vi "novo_config_adq.vi"() -> ()   [LabVIEW 2019]
uses:
  Aplicacao_atual_global_adq.vi
  <vilib>/Utility/file.llb/Write Delimited Spreadsheet (DBL).vi
panel:
  in  "SKM-AI-KF_COR":bool
  in  "SKM-FIC-KF_COR":bool
  in  "SKM-FI-WF":bool
  in  "JG":bool
  in  "JK":bool
  in  "JW":bool
  out "path":path
  in  "SALVAR":bool
  in  "Pfundo":bool
  in  "P4":bool
  in  "P3":bool
  in  "P2":bool
  in  "P1":bool
  in  "C4-M":bool
  in  "C4-J":bool
  in  "C3-J":bool
  in  "C3-M":bool
  in  "C2-J":bool
  in  "C2-M":bool
  in  "C1-J":bool
  in  "C1-M":bool
  # "NOVA CONFIGURACAO PARA O ADQUIRI"
  # "Selecione todos os Instrumento/Valores que deseja trabalhar e salvar no adquiri"
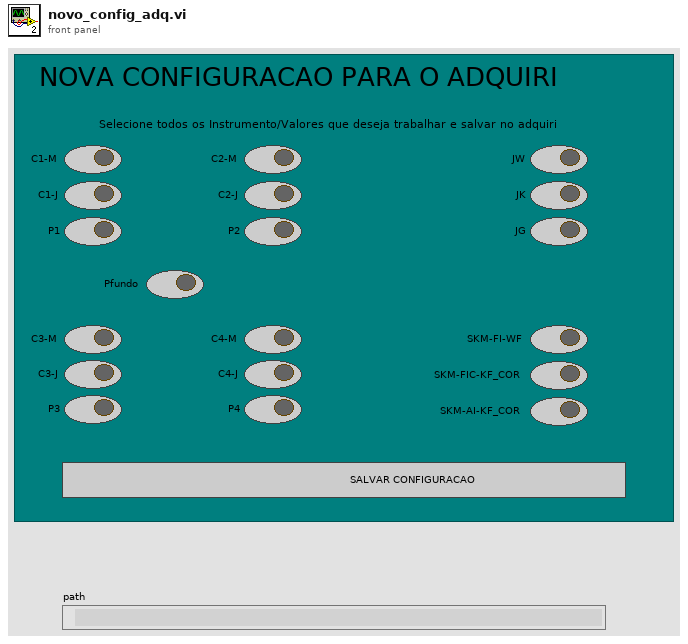
[diagram p1: front panel]
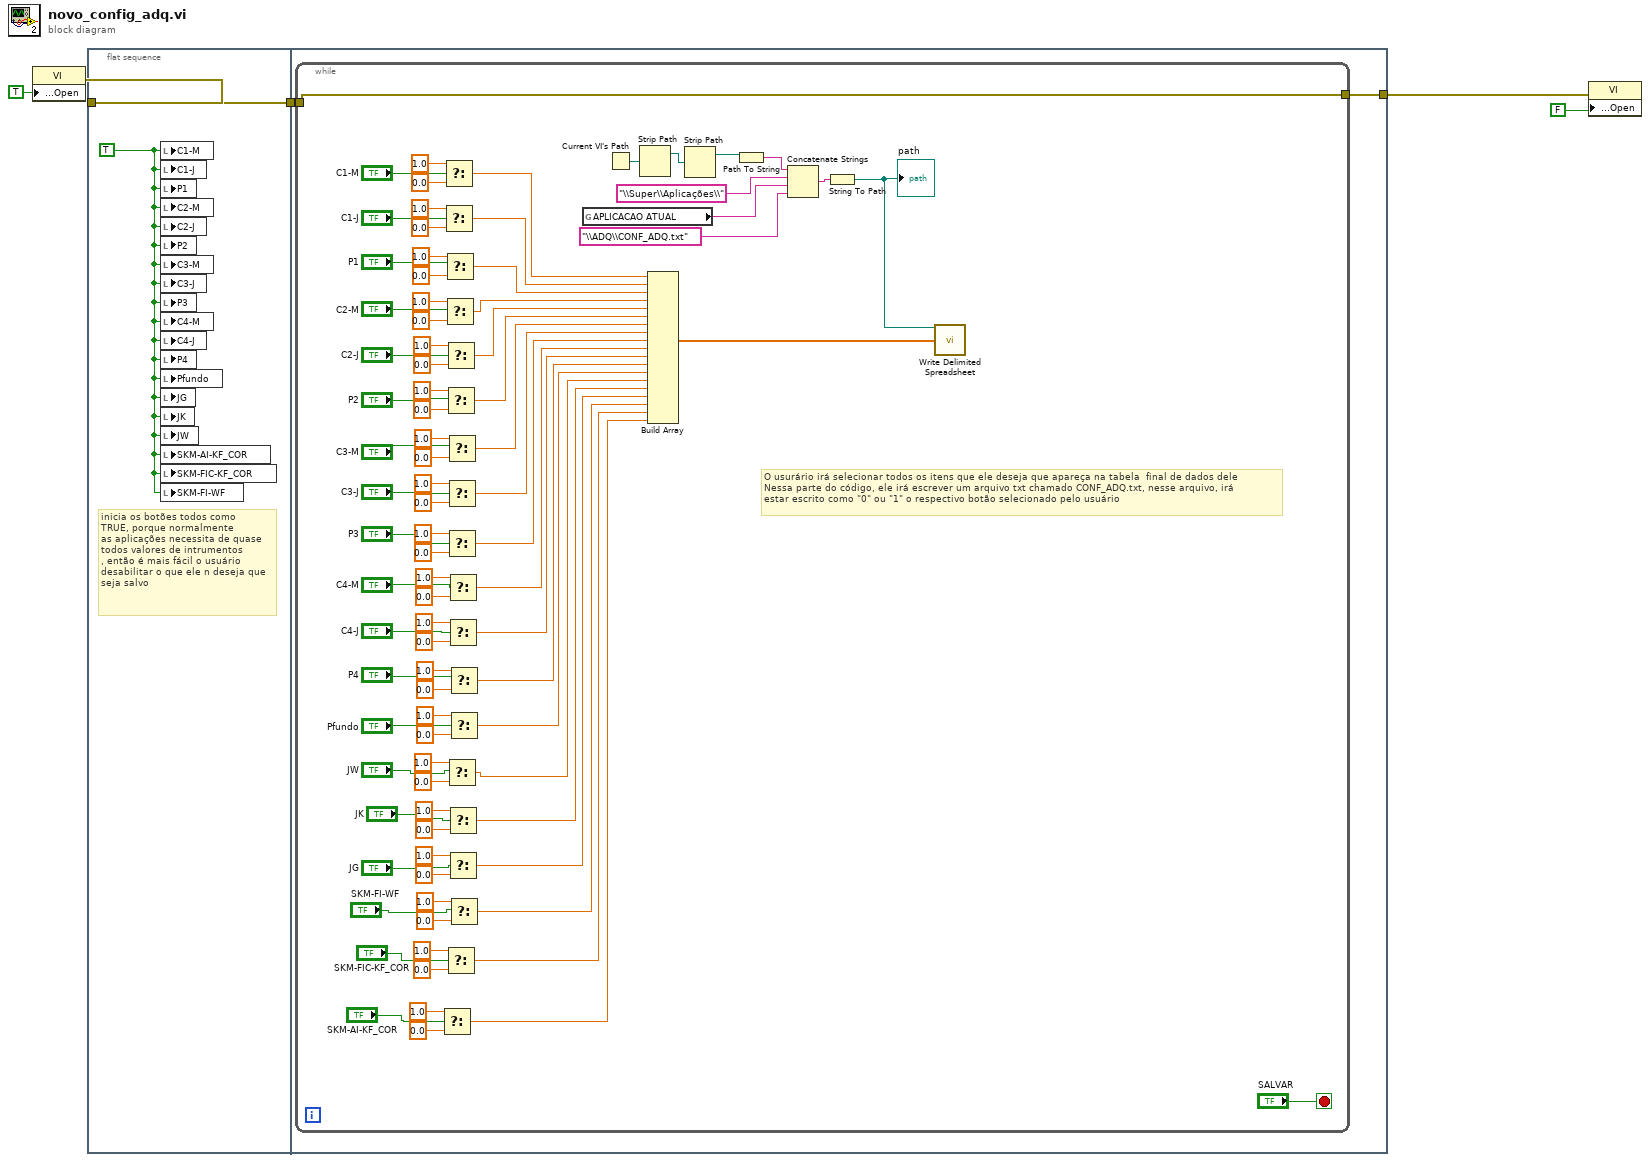
[diagram p0: block diagram]
diagram:
  n1 = property class="VI"("Front Panel.Open"=TRUE ("Front Panel Window:Open")) -> (error out=w3:errorcluster)  [unwired: 2 in, 1 out]
  n2 = flat-sequence {
    tunnel: w3 -> [w7]
    tunnel: [w7] -> w2
    tunnel: w2 -> [w8]
    tunnel: [w9] -> w5
    frame #0 {
      w6 = TRUE ("C1-M")
      # "inicia os botões todos como\nTRUE, porque normalmente\nas aplicações necessita de quase\ntodos valores de intrumentos\n, então é mais fácil o usuário \ndesabilitar o que ele n deseja que\nseja salvo"
      n3 = local write "C1-M"(w6) -> ()
      n4 = local write "C1-J"(w6) -> ()
      n5 = local write "P1"(w6) -> ()
      n6 = local write "C2-M"(w6) -> ()
      n7 = local write "C2-J"(w6) -> ()
      n8 = local write "P2"(w6) -> ()
      n9 = local write "C3-M"(w6) -> ()
      n10 = local write "C3-J"(w6) -> ()
      n11 = local write "P3"(w6) -> ()
      n12 = local write "C4-M"(w6) -> ()
      n13 = local write "C4-J"(w6) -> ()
      n14 = local write "P4"(w6) -> ()
      n15 = local write "Pfundo"(w6) -> ()
      n16 = local write "JG"(w6) -> ()
      n17 = local write "JK"(w6) -> ()
      n18 = local write "JW"(w6) -> ()
      n19 = local write "SKM-AI-KF_COR"(w6) -> ()
      n20 = local write "SKM-FIC-KF_COR"(w6) -> ()
      n21 = local write "SKM-FI-WF"(w6) -> ()
    }
    frame #1 {
      n22 = while {
        tunnel: w8 -> [w24]
        tunnel: [w24] -> w9
        stop <- "SALVAR" stop-if-true
        # "O usurário irá selecionar todos os itens que ele deseja que apareça na tabela  final de dados dele\nNessa parte do código, ele irá escrever um arquivo txt chamado CONF_ADQ.txt, nesse arquivo, irá \nestar escrito como \"0\" ou \"1\" o respectivo botão selecionado pelo usuário"
        n23 = Select(t=1.0, s="SKM-AI-KF_COR", f=0.0) -> (s? t:f=w10:dbl)
        n24 = Select(t=1.0, s="C1-M", f=0.0) -> (s? t:f=w66:dbl)
        n25 = Select(t=1.0, s="C1-J", f=0.0) -> (s? t:f=w65:dbl)
        n26 = Select(t=1.0, s="P1", f=0.0) -> (s? t:f=w64:dbl)
        n27 = Select(t=1.0, s="C2-M", f=0.0) -> (s? t:f=w63:dbl)
        n28 = Select(t=1.0, s="C2-J", f=0.0) -> (s? t:f=w62:dbl)
        n29 = Select(t=1.0, s="P2", f=0.0) -> (s? t:f=w61:dbl)
        n30 = Select(t=1.0, s="SKM-FIC-KF_COR", f=0.0) -> (s? t:f=w11:dbl)
        n31 = Select(t=1.0, s="C3-M", f=0.0) -> (s? t:f=w60:dbl)
        n32 = Select(t=1.0, s="C3-J", f=0.0) -> (s? t:f=w59:dbl)
        n33 = Select(t=1.0, s="P3", f=0.0) -> (s? t:f=w58:dbl)
        n34 = Select(t=1.0, s="JW", f=0.0) -> (s? t:f=w36:dbl)
        n35 = Select(t=1.0, s="C4-M", f=0.0) -> (s? t:f=w57:dbl)
        n36 = Select(t=1.0, s="C4-J", f=0.0) -> (s? t:f=w56:dbl)
        n37 = Select(t=1.0, s="JK", f=0.0) -> (s? t:f=w34:dbl)
        n38 = Select(t=1.0, s="JG", f=0.0) -> (s? t:f=w35:dbl)
        n39 = Select(t=1.0, s="P4", f=0.0) -> (s? t:f=w55:dbl)
        n40 = Select(t=1.0, s="Pfundo", f=0.0) -> (s? t:f=w54:dbl)
        n41 = Select(t=1.0, s="SKM-FI-WF", f=0.0) -> (s? t:f=w12:dbl)
        n42 = global read "Aplicacao_atual_global_adq.vi" "APLICACAO ATUAL"() -> (w45:string)
        n43 = Current VI's Path() -> (path=w51:path)
        n44 = Strip Path(path=w51) -> (stripped path=w47:path)  [unwired: 1 out]
        n45 = Build Array(w66, w65, w64, w63, w62, w61, w60, w59, w58, w57, w56, w55, w54, w36, w34, w35, w12, w11, w10) -> (w53:dbl[])
        n46 = Strip Path(path=w47) -> (stripped path=w46:path)  [unwired: 1 out]
        n47 = Path To String(path=w46) -> (string=w52:string)
        n48 = Concatenate Strings(w52, "\\Super\\Aplicações\\" ("string"), w45, "\\ADQ\\CONF_ADQ.txt" ("string")) -> (w49:string)
        n49 = String To Path(string=w49) -> (path=w48:path)
        "path" <- w48
        n50 = call-poly <vilib>:"Write Delimited Spreadsheet.vi"("file path (dialog if empty)"=w48, "1D data"=w53) -> ()  [unwired: 12 in, 2 out]
      }
    }
  }
  n51 = property class="VI"(error in=w5, "Front Panel.Open"=FALSE ("Front Panel Window:Open")) -> ()  [unwired: 1 in, 2 out]
